vi "RS232发送接收.vi"() -> ()   [LabVIEW 2010]
uses:
  <vilib>/Instr/_visa.llb/VISA Configure Serial Port (Instr).vi
panel:
  out "接收数据_2":string
  out "成功_2？":bool caption="成功？"
  in  "发送数据_2":string
  in  "btn_关闭":bool
  in  "btn_开始测试":bool
  out "接收数据_1":string
  out "成功_1？":bool caption="成功？"
  in  "发送数据_1":string
  # "RS232测试界面"
  # "1#发送字符"
  # "2#发送字符"
  # "1#接收字符"
  # "2#接收字符"
  # "1#测试结果"
  # "2#测试结果"
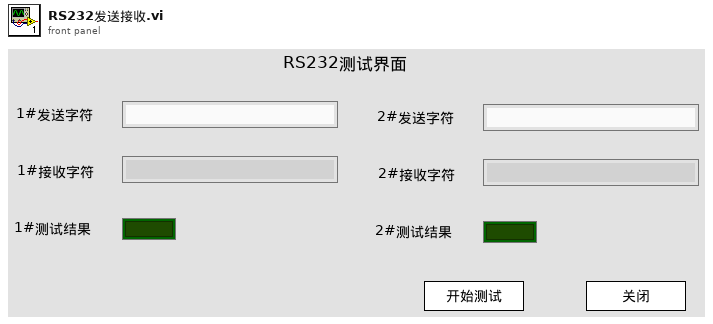
[diagram p1: front panel]
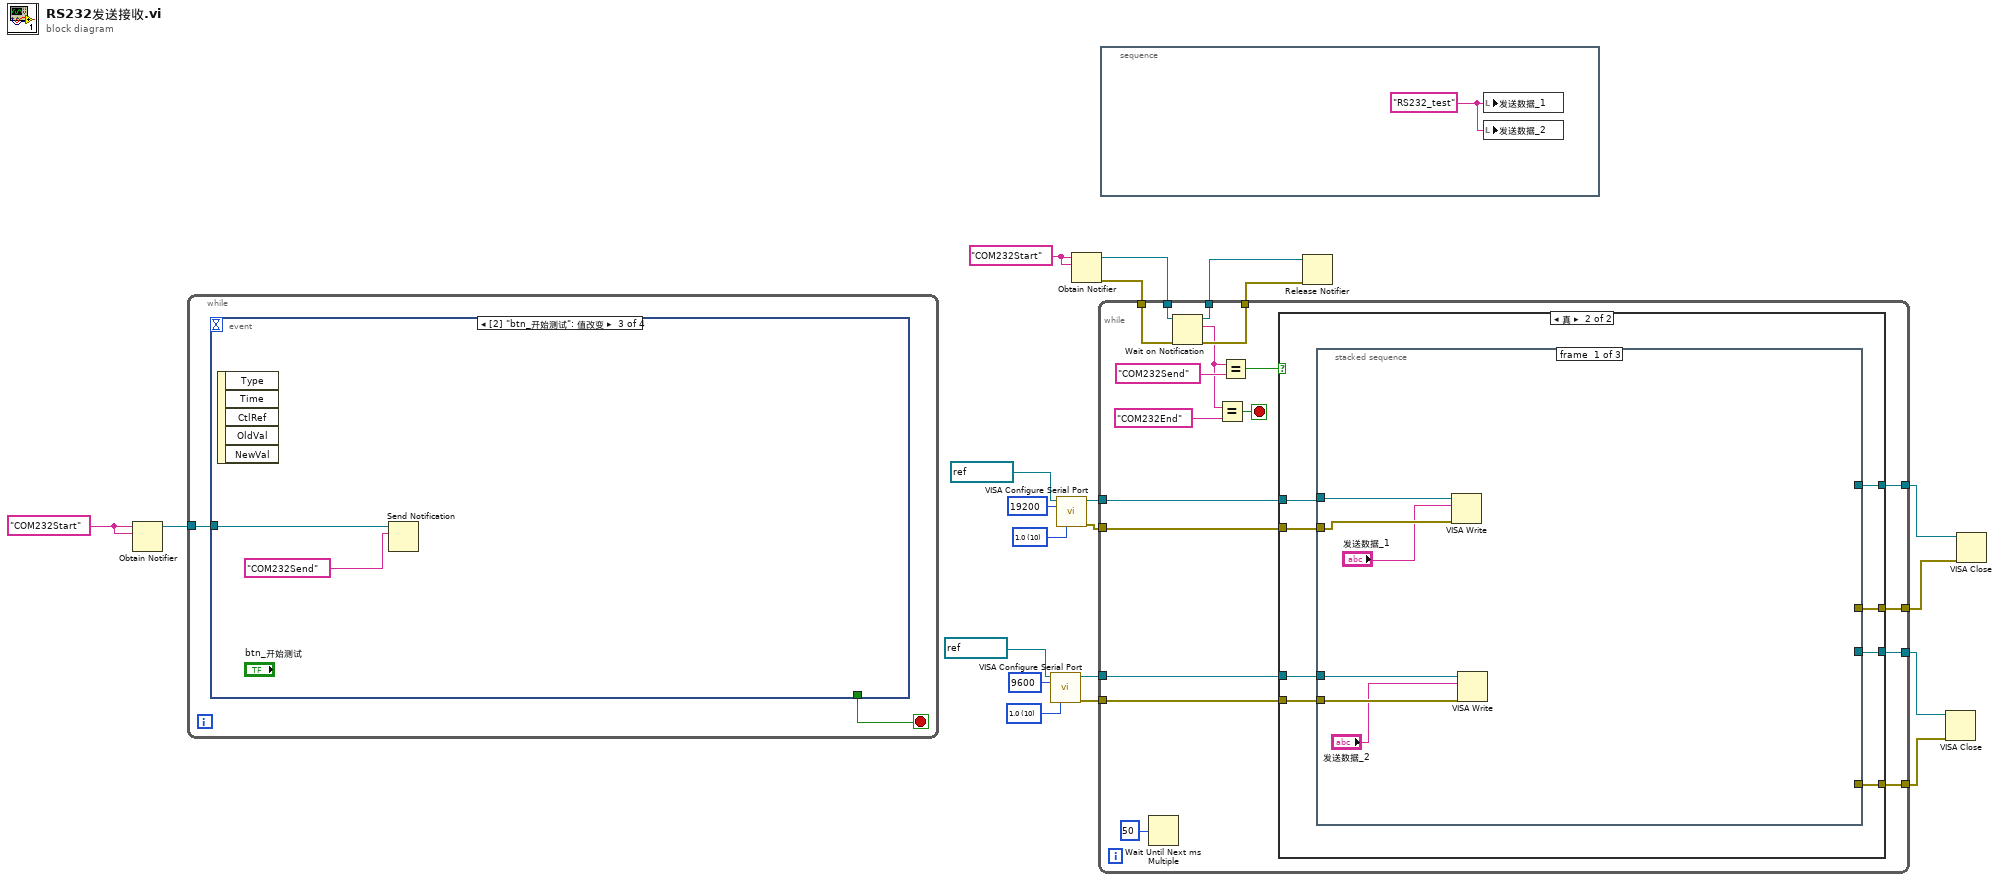
[diagram p0: block diagram]
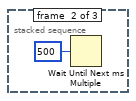
[diagram p3: hidden frame]
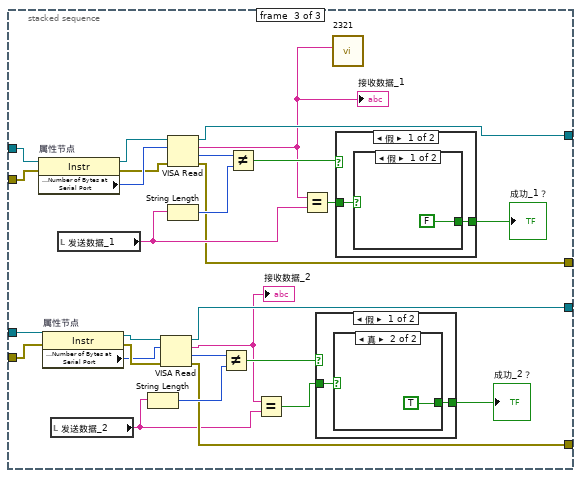
[diagram p4: hidden frame]
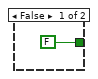
[diagram p5: hidden frame]
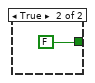
[diagram p6: hidden frame]
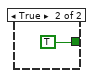
[diagram p7: hidden frame]
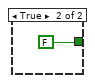
[diagram p8: hidden frame]
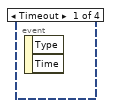
[diagram p9: hidden frame]
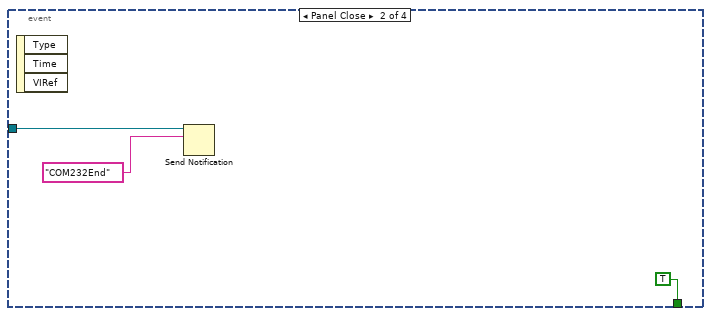
[diagram p10: hidden frame]
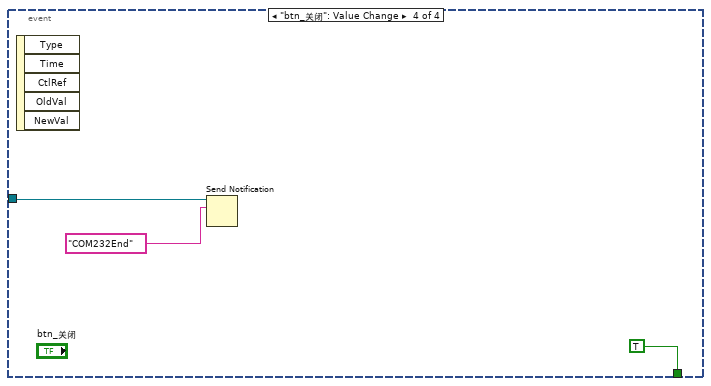
[diagram p11: hidden frame]
diagram:
  w5 = u16 10 items=["1.0"=10, "1.5"=15, "2.0"=20] ("stop bits (10: 1 bit)")
  w11 = "COM232Start" ("名称（未命名）")
  w20 = "COM232Start" ("名称（未命名）")
  w21 = u16 10 items=["1.0"=10, "1.5"=15, "2.0"=20] ("stop bits (10: 1 bit)")
  n1 = Obtain Notifier(name (unnamed)=w11, notification data type=w11) -> (notifier out=w10:refnum<notifier>)  [unwired: 2 in, 2 out]
  n2 = while {
    tunnel: w10 -> [w22]
    stop <- w23 stop-if-true
    n3 = event shown="[2] \"btn_开始测试\": 值改变" {
      selector: _ -> [_ _ _ _]
      dyn-events: _ -> [_ _ _ _]
      timeout: _ -> [_ _ _ _]
      tunnel: [_ TRUE _ TRUE] -> w23
      tunnel: w22 -> [_ w25 w27 w29]
      event Timeout {
        n4 = event-data() -> ()  [unwired: 1 in, 2 out]
      }
      event Panel Close {
        n5 = event-data() -> ()  [unwired: 1 in, 3 out]
        n6 = Send Notification(notification="COM232End" ("通知"), notifier=w25) -> ()  [unwired: 1 in, 2 out]
      }
      event "btn_开始测试": Value Change {
        n7 = event-data() -> ()  [unwired: 1 in, 5 out]
        n8 = Send Notification(notification="COM232Send" ("通知"), notifier=w27) -> ()  [unwired: 1 in, 2 out]
      }
      event "btn_关闭": Value Change {
        n9 = event-data() -> ()  [unwired: 1 in, 5 out]
        n10 = Send Notification(notification="COM232End" ("通知"), notifier=w29) -> ()  [unwired: 1 in, 2 out]
      }
    }
  }
  n11 = call-poly "VISA Configure Serial Port"("VISA resource name"=refnum<visa-resource-name> "COM3" ("R232端口"), "baud rate (9600)"=u32 9600, "stop bits (10: 1 bit)"=w5) -> ("VISA resource name out"=w4:refnum<visa-resource-name>, "error out"=w3:errorcluster)  [unwired: 11 in]
  n12 = call-poly "VISA Configure Serial Port"("VISA resource name"=refnum<visa-resource-name> "COM1" ("R232端口"), "baud rate (9600)"=u32 19200, "stop bits (10: 1 bit)"=w21) -> ("VISA resource name out"=w15:refnum<visa-resource-name>, "error out"=w14:errorcluster)  [unwired: 11 in]
  n13 = Obtain Notifier(name (unnamed)=w20, notification data type=w20) -> (notifier out=w19:refnum<notifier>, error out=w18:errorcluster)  [unwired: 2 in, 1 out]
  n14 = while {
    tunnel: w19 -> [w49]
    tunnel: w18 -> [w48]
    tunnel: [w47] -> w17
    tunnel: [w46] -> w16
    tunnel: w15 -> [w43]
    tunnel: w14 -> [w42]
    tunnel: [w41] -> w13
    tunnel: [w40] -> w12
    tunnel: w4 -> [w35]
    tunnel: w3 -> [w34]
    tunnel: [w33] -> w2
    tunnel: [w32] -> w1
    stop <- w37 stop-if-true
    n15 = Wait Until Next ms Multiple(millisecond multiple=u32 50 ("毫秒倍数")) -> ()  [unwired: 1 out]
    n16 = Wait on Notification(notifier=w49, error in (no error)=w48) -> (notifier out=w47:refnum<notifier>, notification=w39:string, error out=w46:errorcluster)  [unwired: 2 in, 1 out]
    n17 = Equal?(x=w39, y="COM232End" ("通知")) -> (x = y?=w37:bool)
    n18 = Equal?(x=w39, y="COM232Send" ("通知")) -> (x = y?=w44:bool)
    n19 = case shown="真" w44 {
      tunnel: w43 -> [w53 w61]
      tunnel: w42 -> [w52 w60]
      tunnel: [w53 w59] -> w41
      tunnel: [w52 w58] -> w40
      tunnel: w35 -> [w51 w57]
      tunnel: w34 -> [w50 w56]
      tunnel: [w51 w55] -> w33
      tunnel: [w50 w54] -> w32
      frame False {
      }
      frame True {
        n20 = stacked-sequence {
          tunnel: w61 -> [w67 _ w85]
          tunnel: w60 -> [w66 _ w84]
          tunnel: [_ _ w87] -> w59
          tunnel: [_ _ w86] -> w58
          tunnel: w57 -> [w64 _ w83]
          tunnel: w56 -> [w63 _ w82]
          tunnel: [_ _ w76] -> w55
          tunnel: [_ _ w75] -> w54
          frame #0 {
            n21 = VISA Write(VISA resource name=w67, write buffer="发送数据_1", error in (no error)=w66) -> ()  [unwired: 3 out]
            n22 = VISA Write(VISA resource name=w64, write buffer="发送数据_2", error in (no error)=w63) -> ()  [unwired: 3 out]
          }
          frame #1 {
            n23 = Wait Until Next ms Multiple(millisecond multiple=u32 500 ("毫秒倍数")) -> ()  [unwired: 1 out]
          }
          frame #2 {
            n24 = property on="属性节点" class="Instr"(reference=w85, error in=w84) -> (reference out=w94:refnum<visa-resource-name>, error out=w92:errorcluster, "Serial Settings:Number of Bytes at Serial Port"=w93:u32)
            n25 = property on="属性节点" class="Instr"(reference=w83, error in=w82) -> (reference out=w81:refnum<visa-resource-name>, error out=w80:errorcluster, "Serial Settings:Number of Bytes at Serial Port"=w79:u32)
            n26 = local read "发送数据_2"() -> (w73:string)
            n27 = local read "发送数据_1"() -> (w91:string)
            n28 = String Length(string=w73) -> (length=w78:i32)
            n29 = VISA Read(VISA resource name=w81, byte count=w79, error in (no error)=w80) -> (VISA resource name out=w76:refnum<visa-resource-name>, read buffer=w70:string, return count=w77:u32, error out=w75:errorcluster)
            "接收数据_2" <- w70
            n30 = VISA Read(VISA resource name=w94, byte count=w93, error in (no error)=w92) -> (VISA resource name out=w87:refnum<visa-resource-name>, read buffer=w69:string, return count=w90:u32, error out=w86:errorcluster)
            "接收数据_1" <- w69
            n31 = String Length(string=w91) -> (length=w89:i32)
            n32 = Not Equal?(x=w77, y=w78) -> (x != y?=w74:bool)
            n33 = Not Equal?(x=w90, y=w89) -> (x != y?=w88:bool)
            n34 = Equal?(x=w70, y=w73) -> (x = y?=w72:bool)
            n35 = Equal?(x=w69, y=w91) -> (x = y?=w96:bool)
            n36 = case shown="假" w74 {
              tunnel: w72 -> [w98 _]
              tunnel: [w97 FALSE] -> w71
              frame False {
                n37 = case shown="真" w98 {
                  tunnel: [FALSE TRUE] -> w97
                  frame False {
                  }
                  frame True {
                  }
                }
              }
              frame True {
              }
            }
            "成功_2？" <- w71
            n38 = call "2321"("Message"=w69) -> ()  [unwired: 9 in, 2 out]
            n39 = case shown="假" w88 {
              tunnel: w96 -> [w103 _]
              tunnel: [w102 FALSE] -> w95
              frame False {
                n40 = case shown="假" w103 {
                  tunnel: [FALSE TRUE] -> w102
                  frame False {
                  }
                  frame True {
                  }
                }
              }
              frame True {
              }
            }
            "成功_1？" <- w95
          }
        }
      }
    }
  }
  n41 = stacked-sequence {
    frame #0 {
      w107 = "RS232_test" ("发送数据_1")
      n42 = local write "发送数据_1"(w107) -> ()
      n43 = local write "发送数据_2"(w107) -> ()
    }
  }
  n44 = Release Notifier(notifier=w17, error in (no error)=w16) -> ()  [unwired: 1 in, 3 out]
  n45 = VISA Close(VISA resource name=w2, error in (no error)=w1) -> ()  [unwired: 1 out]
  n46 = VISA Close(VISA resource name=w13, error in (no error)=w12) -> ()  [unwired: 1 out]
